vi "Logger.vi"(7 "Action":T1, 8 "Error In":errorcluster, 11 "Message":string) -> (0 "Error Out":errorcluster, 3 "Event":refnum<user-event>)   [LabVIEW 2014, in "LV-Logger.lvlib"]
uses:
  LV-Logger.lvlib
  Action.ctl
  Log.ctl
  Level.ctl
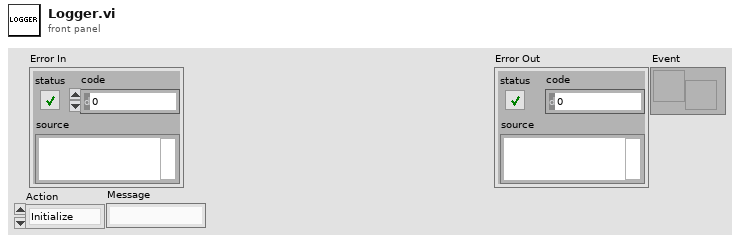
[diagram p1: front panel]
types:
  T1 = typedef "LV-Logger.lvlib/Action.ctl" = enum16{"Initialize", "Get", "Fatal", "Error", "Debug", "Warn", "Info", "Trace", "Shutdown"}
  T2 = typedef "LV-Logger.lvlib/Log.ctl" = cluster{"Level":T3, "Source":string, "Message":string}
  T3 = typedef "LV-Logger.lvlib/Level.ctl" = enum16{"Fatal", "Error", "Warn", "Debug", "Info", "Trace"}
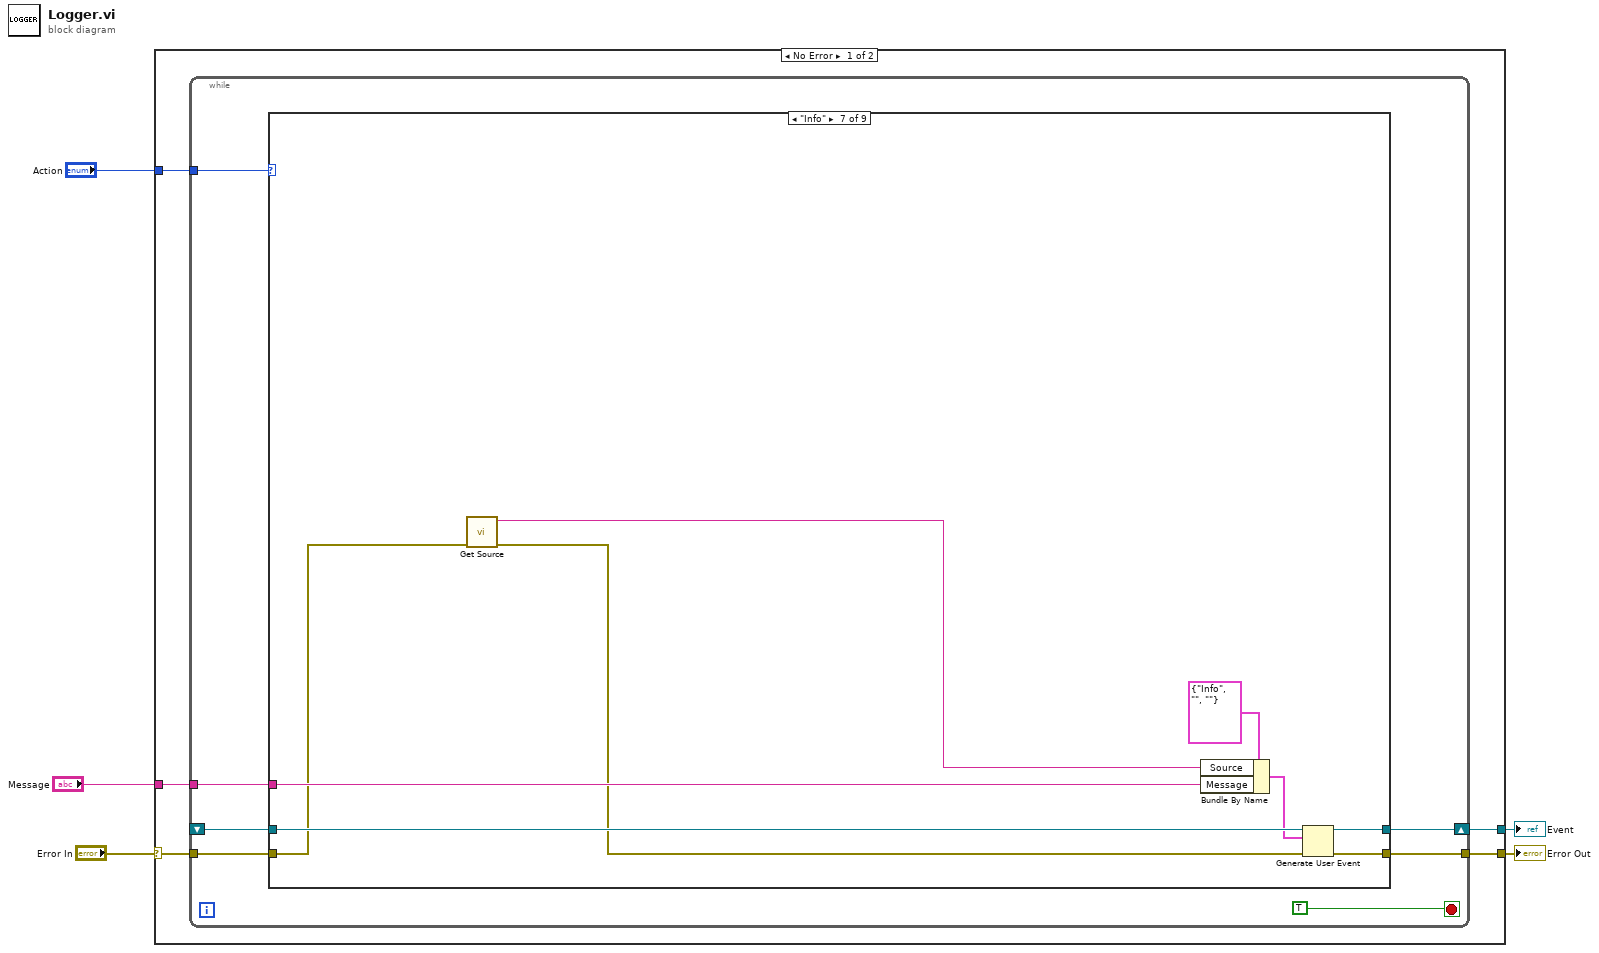
[diagram p0: block diagram]
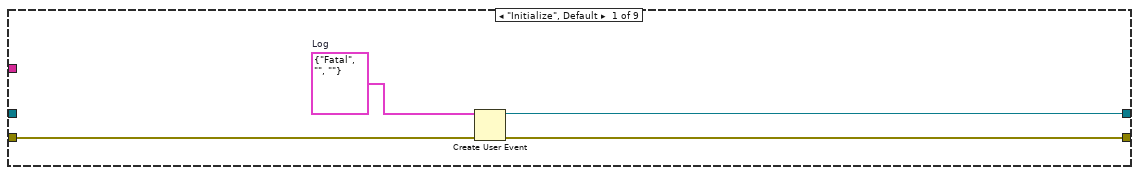
[diagram p2: hidden frame]
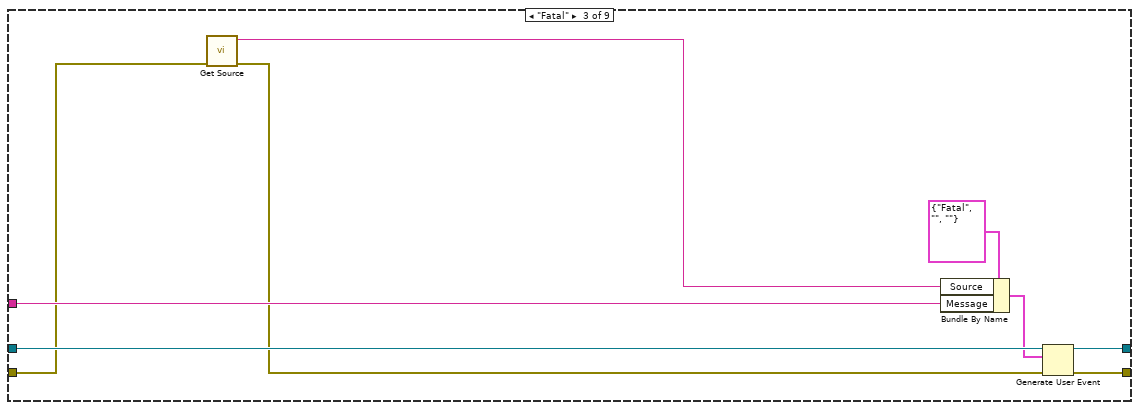
[diagram p4: hidden frame]
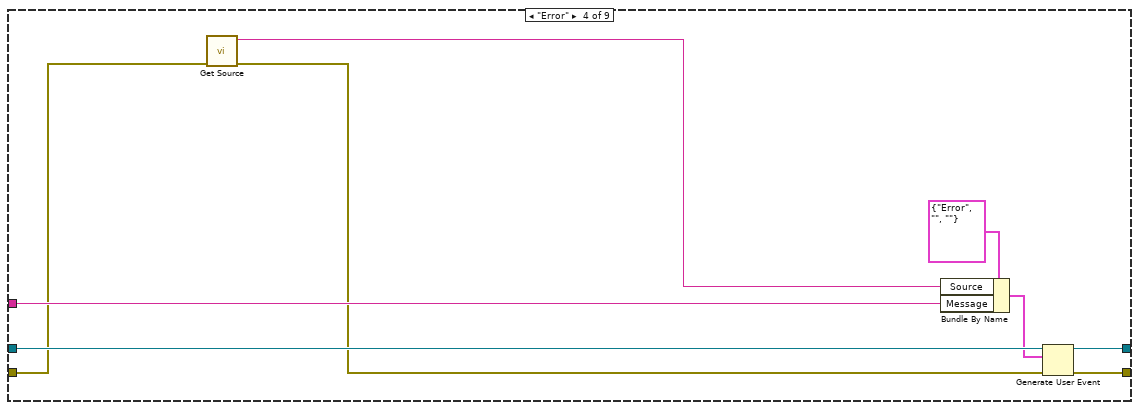
[diagram p5: hidden frame]
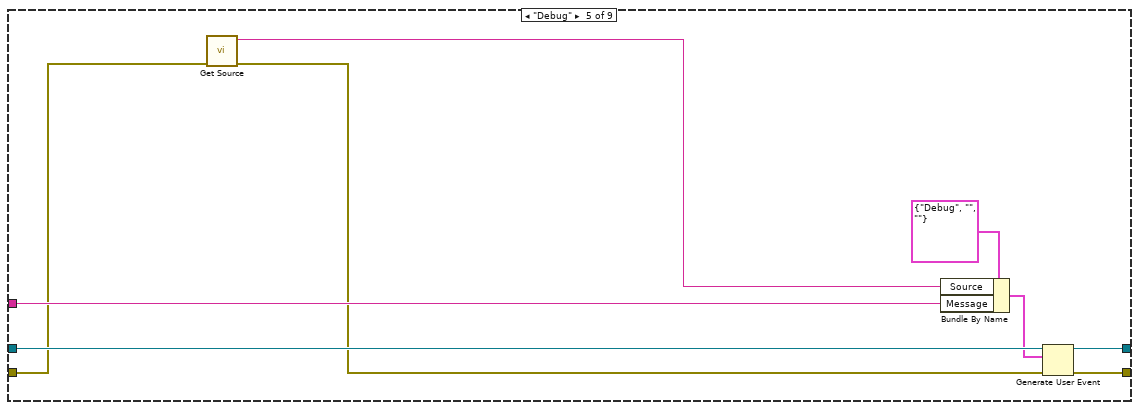
[diagram p6: hidden frame]
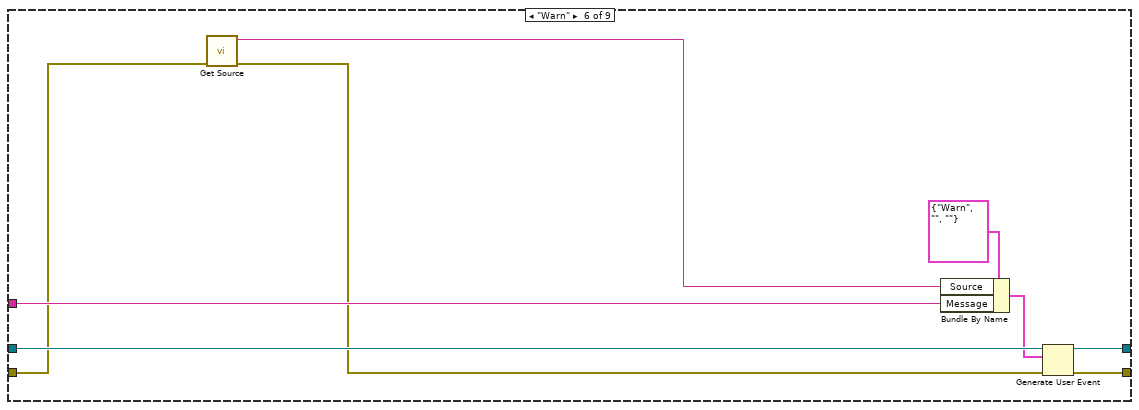
[diagram p7: hidden frame]
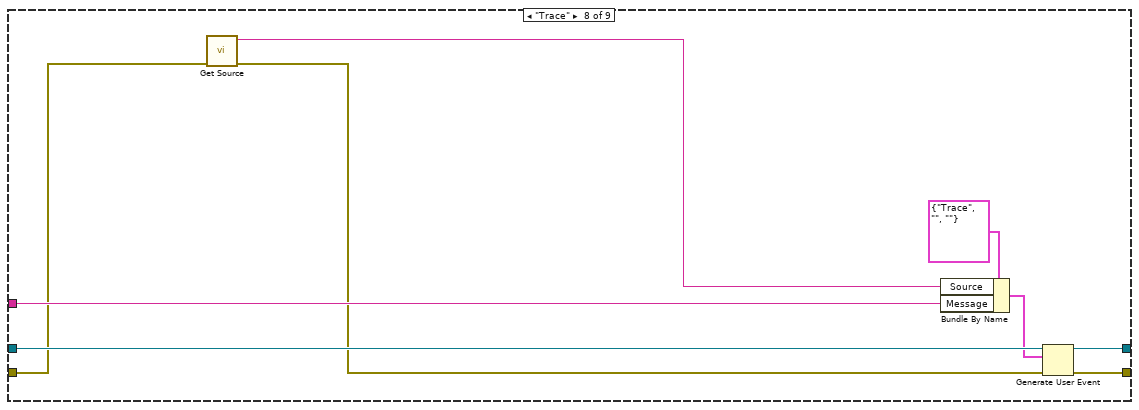
[diagram p8: hidden frame]
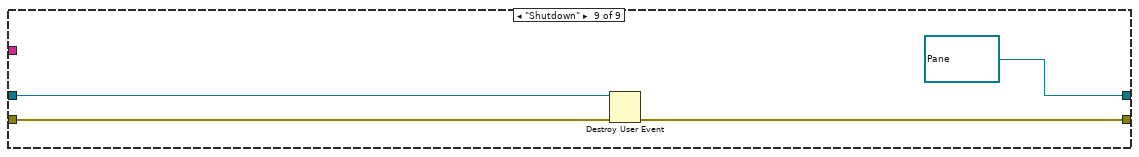
[diagram p9: hidden frame]
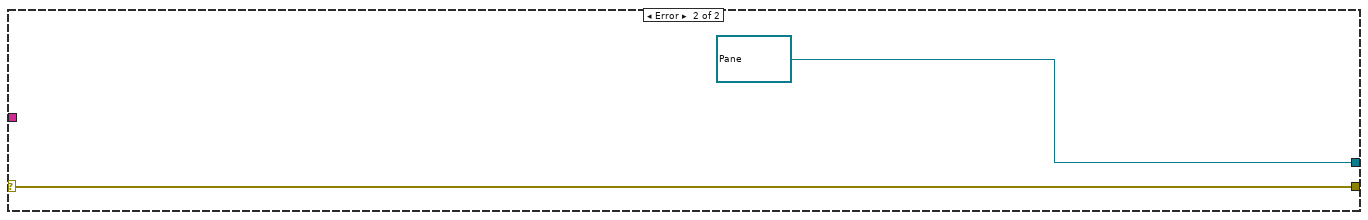
[diagram p10: hidden frame]
diagram:
  n1 = case shown="No Error" "Error In" {
    selector: "Error In" -> [w9 w83]
    tunnel: [w8 w83] -> w4
    tunnel: "Action" -> [w10 _]
    tunnel: [w7 refnum<user-event> refnum ("Log")] -> w1
    tunnel: "Message" -> [w6 _]
    frame No Error {
      n2 = while {
        tunnel: w10 -> [w16]
        tunnel: w9 -> [w15]
        tunnel: [w14] -> w8
        shift-right: [w13] -> w7
        shift-left: _ -> [w12]
        tunnel: w6 -> [w11]
        stop <- TRUE stop-if-true
        n3 = case shown="\"Info\"" w16 {
          tunnel: w15 -> [w21 w23 w25 w34 w43 w52 w61 w70 w81]
          tunnel: [w20 w23 w30 w39 w48 w57 w66 w75 w79] -> w14
          tunnel: [w19 w22 w31 w40 w49 w58 w67 w76 refnum<user-event> refnum ("Log")] -> w13
          tunnel: w12 -> [_ w22 w32 w41 w50 w59 w68 w77 w80]
          tunnel: w11 -> [_ _ w27 w36 w45 w54 w63 w72 _]
          frame "Initialize", Default {
            w18 = T2 {"Level"=enum."Fatal", "Source"="", "Message"=""}  # Log
            n4 = Create User Event(user event datatype=w18, error in=w21) -> (user event=w19:refnum<user-event>, error out=w20:errorcluster)
          }
          frame "Get" {
          }
          frame "Fatal" {
            n5 = call "Get Source.vi"("Error In"=w25) -> ("Error Out"=w24:errorcluster, "Source"=w26:string)  [unwired: 9 in]
            n6 = Bundle By Name(cluster=T2 {"Level"=enum."Fatal", "Source"="", "Message"=""} ("event data"), "Source"=w26, "Message"=w27) -> (w28:T2)
            n7 = Generate User Event(user event=w32, event data cluster=w28, error in=w24) -> (user event out=w31:refnum<user-event>, error out=w30:errorcluster)  [unwired: 1 in]
          }
          frame "Error" {
            n8 = call "Get Source.vi"("Error In"=w34) -> ("Error Out"=w33:errorcluster, "Source"=w35:string)  [unwired: 9 in]
            n9 = Bundle By Name(cluster=T2 {"Level"=enum."Error", "Source"="", "Message"=""} ("event data"), "Source"=w35, "Message"=w36) -> (w37:T2)
            n10 = Generate User Event(user event=w41, event data cluster=w37, error in=w33) -> (user event out=w40:refnum<user-event>, error out=w39:errorcluster)  [unwired: 1 in]
          }
          frame "Debug" {
            n11 = call "Get Source.vi"("Error In"=w43) -> ("Error Out"=w42:errorcluster, "Source"=w44:string)  [unwired: 9 in]
            n12 = Bundle By Name(cluster=T2 {"Level"=enum."Debug", "Source"="", "Message"=""} ("event data"), "Source"=w44, "Message"=w45) -> (w46:T2)
            n13 = Generate User Event(user event=w50, event data cluster=w46, error in=w42) -> (user event out=w49:refnum<user-event>, error out=w48:errorcluster)  [unwired: 1 in]
          }
          frame "Warn" {
            n14 = call "Get Source.vi"("Error In"=w52) -> ("Error Out"=w51:errorcluster, "Source"=w53:string)  [unwired: 9 in]
            n15 = Bundle By Name(cluster=T2 {"Level"=enum."Warn", "Source"="", "Message"=""} ("event data"), "Source"=w53, "Message"=w54) -> (w55:T2)
            n16 = Generate User Event(user event=w59, event data cluster=w55, error in=w51) -> (user event out=w58:refnum<user-event>, error out=w57:errorcluster)  [unwired: 1 in]
          }
          frame "Info" {
            n17 = call "Get Source.vi"("Error In"=w61) -> ("Error Out"=w60:errorcluster, "Source"=w62:string)  [unwired: 9 in]
            n18 = Bundle By Name(cluster=T2 {"Level"=enum."Info", "Source"="", "Message"=""} ("event data"), "Source"=w62, "Message"=w63) -> (w64:T2)
            n19 = Generate User Event(user event=w68, event data cluster=w64, error in=w60) -> (user event out=w67:refnum<user-event>, error out=w66:errorcluster)  [unwired: 1 in]
          }
          frame "Trace" {
            n20 = call "Get Source.vi"("Error In"=w70) -> ("Error Out"=w69:errorcluster, "Source"=w71:string)  [unwired: 9 in]
            n21 = Bundle By Name(cluster=T2 {"Level"=enum."Trace", "Source"="", "Message"=""} ("event data"), "Source"=w71, "Message"=w72) -> (w73:T2)
            n22 = Generate User Event(user event=w77, event data cluster=w73, error in=w69) -> (user event out=w76:refnum<user-event>, error out=w75:errorcluster)  [unwired: 1 in]
          }
          frame "Shutdown" {
            n23 = Destroy User Event(user event=w80, error in=w81) -> (error out=w79:errorcluster)
          }
        }
      }
    }
    frame Error {
    }
  }
  "Error Out" <- w4
  "Event" <- w1
